vi "conversionsTempEth.vi"(5 "Array":dbl[](array[numeric]), 8 "error in (no error)":errorcluster, 11 "Parameters":T1={"RH/T Sensor VSS (V)"=5.048, "K0"=0.9054, "K1"=-2.995, "Offset"=0.0, "Gain"=1.0, "Samples/Channel/s"=1000.0, "Samples to Average"=100.0} {"Offset" step=0.01 format="%_3f"; "K1" format="%#_13g"; "K0" format="%#_13g"; "RH/T Sensor VSS (V)" format="%.3g"}) -> (0 "error out":errorcluster, 1 "T":dbl, 2 "RH":dbl, 3 "Ethanol":dbl)   [LabVIEW 2020]
uses:
  typeDefs/Parameters.ctl
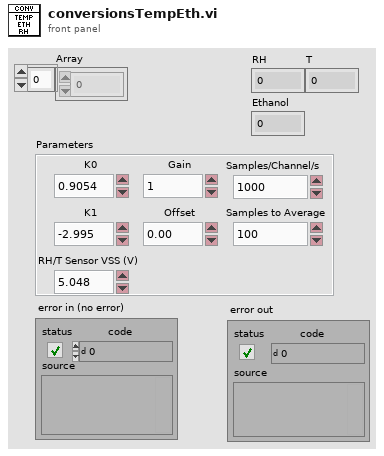
[diagram p1: front panel]
types:
  T1 = typedef "Parameters.ctl" = cluster{"RH/T Sensor VSS (V)":dbl, "K0":dbl, "K1":dbl, "Offset":dbl, "Gain":dbl, "Samples/Channel/s":dbl, "Samples to Average":dbl}
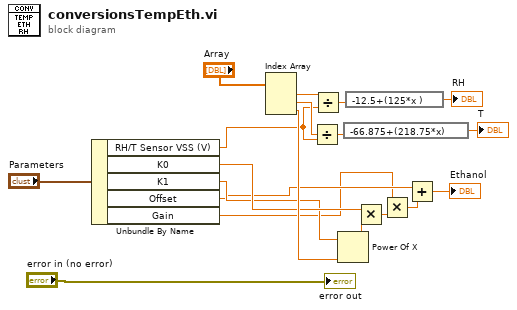
[diagram p0: block diagram]
diagram:
  n1 = Unbundle By Name("Parameters") -> ("RH/T Sensor VSS (V)"=w5:dbl, "K0"=w4:dbl, "K1"=w3:dbl, "Offset"=w2:dbl, "Gain"=w1:dbl)
  n2 = Index Array(array="Array") -> (element #1=w12:dbl, element #2=w13:dbl, element #3=w19:dbl)  [unwired: 3 in]
  n3 = Divide(x=w13, y=w5) -> (x/y=w15:dbl)
  n4 = Divide(x=w12, y=w5) -> (x/y=w14:dbl)
  n5 = Power Of X(1:w19, 2:w3) -> (0:w18:dbl)
  n6 = expression code="-66.875+(218.75*x)"(w15) -> (→"T":dbl)
  n7 = expression code="-12.5+(125*x )"(w14) -> (→"RH":dbl)
  n8 = Multiply(x=w4, y=w18) -> (x*y=w17:dbl)
  n9 = Multiply(x=w1, y=w17) -> (x*y=w16:dbl)
  n10 = Add(x=w2, y=w16) -> (x+y=→"Ethanol":dbl)
  "error out" <- "error in (no error)"
